vi "5-k-invdist.vi"(8 "err in":errorcluster, 9 "F(k)":dbl, 11 "Loi de Poisson":T1 caption="p_POI") -> (0 "err out":errorcluster caption="err  out", 1 "F(k)":dbl, 2 "k":dbl, 3 "Loi de Poisson":T1 caption="p_POI", 5 "k interpolé":dbl)   [LabVIEW 2010, in "lv_02.lvlib"]
uses:
  p_5E5_LPoi.ctl
  <vilib>/gmath/statdist.llb/Poisson Inverse CDF.vi
  lv_02.lvlib
  <vilib>/gmath/NI_Gmath.lvlib
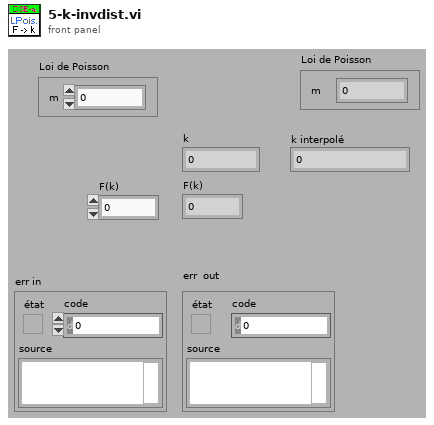
[diagram p1: front panel]
types:
  T1 = typedef "lv_02.lvlib/p_5E5_LPoi.ctl" = cluster{"m":dbl}
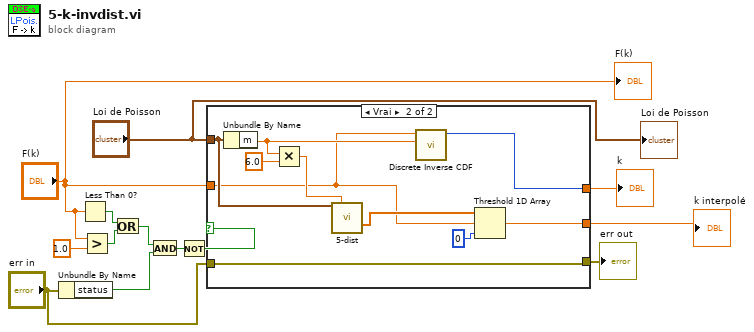
[diagram p0: block diagram]
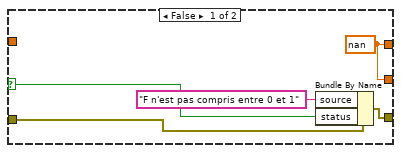
[diagram p2: hidden frame]
diagram:
  n1 = Unbundle By Name("err in") -> ("status"=w7:bool)
  n2 = Less Than 0?(x="F(k)") -> (x < 0?=w9:bool)
  n3 = Greater?(x="F(k)", y=1.0) -> (0:w10:bool)
  n4 = Or(x=w9, y=w10) -> (x .or. y?=w8:bool)
  n5 = And(x=w8, y=w7) -> (x .and. y?=w6:bool)
  n6 = Not(x=w6) -> (.not. x?=w5:bool)
  n7 = case shown="Vrai" w5 {
    selector: w5 -> [w16 _]
    tunnel: "F(k)" -> [_ w19]
    tunnel: [w14 w28] -> w13
    tunnel: "err in" -> [w17 w27]
    tunnel: [w18 w27] -> w3
    tunnel: "Loi de Poisson" -> [_ w20]
    tunnel: [w14 w24] -> w1
    frame False {
      w14 = nan ("x")
      n8 = Bundle By Name(cluster=w17, "source"="F n'est pas compris entre 0 et 1", "status"=w16) -> (w18:errorcluster)
    }
    frame True {
      n9 = Unbundle By Name(w20) -> ("m"=w23:dbl)
      n10 = Multiply(x=w23, y=6.0) -> (x*y=w21:dbl)
      n11 = call "5-dist.vi"("Poisson (m)"=w20, "k max"=w21) -> ("F(0 à k max)"=w25:dbl[])  [unwired: 11 in, 2 out]
      n12 = call-poly <vilib>:"Discrete Inverse CDF.vi"("lambda"=w23, "cdf(x)"=w19) -> ("x"=w28:i32)  [unwired: 8 in, 1 out]
      n13 = Threshold 1D Array(1:0 ("indice de départ (0)"), 2:w19, 3:w25) -> (0:w24:dbl)
    }
  }
  "k" <- w13
  "err out" <- w3
  "k interpolé" <- w1
  "F(k)" <- "F(k)"
  "Loi de Poisson" <- "Loi de Poisson"
